vi "keithley-2450_sweep.vi"(4 "Timeout (ms)":i32=10000000, 5 "Scan direction":u16(ring) items=["Ascending", "Descending"], 6 "Number of Points":u32=5, 7 "End voltage (V)":dbl=2.0, 8 "Start voltage (V)":dbl=1.0, 9 "VISA resource name out 2":refnum<visa-resource-name>) -> (0 "Measurement Complete":bool, 2 "Data Array":dbl[][](array[numeric]), 3 "VISA resource name out":refnum<visa-resource-name>)   [LabVIEW 2016]
doc: "Configures a sweep and takes voltage and current readings at each point."
uses:
  <instrlib>/Keithley 2450/Keithley 2450.lvlib
panel:
  in  "Source Mode  (0: Voltage)":u16(ring) items=["Voltage", "Current"]
  # "(c) 2006 National Instruments.  ALL RIGHTS RESERVED."
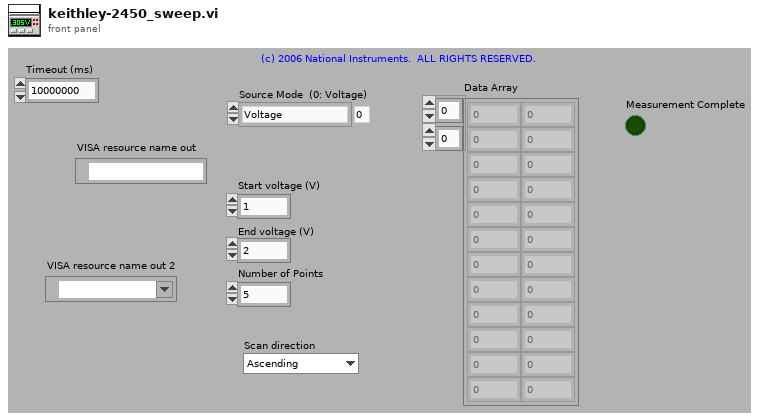
[diagram p1: front panel]
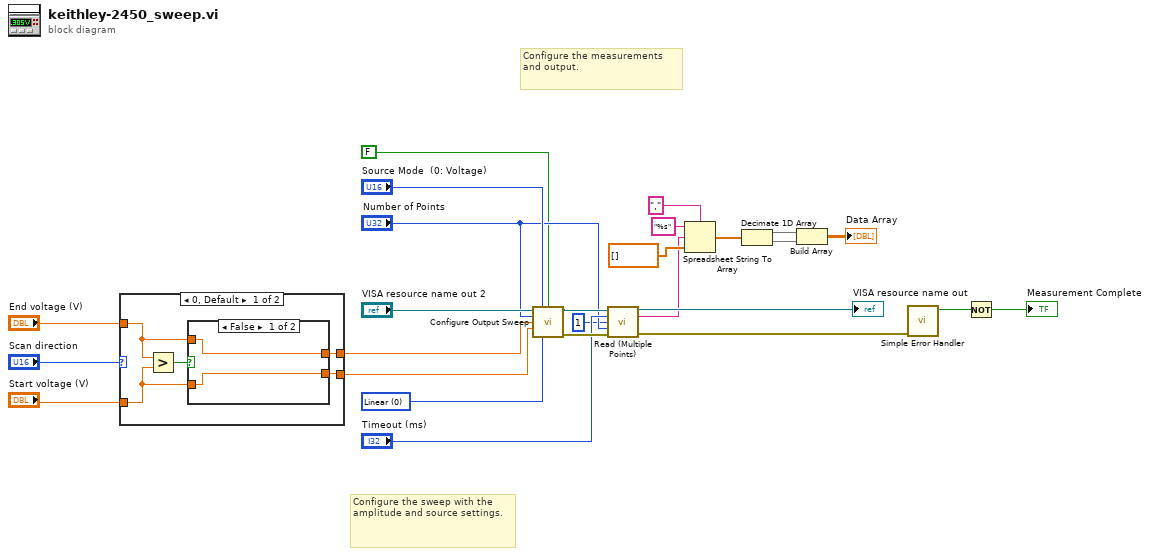
[diagram p0: block diagram]
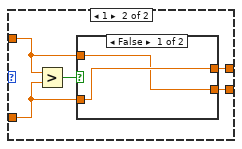
[diagram p3: hidden frame]
diagram:
  w17 = u16 0 items=["Linear", "Logarithmic"] ("Sweep Spacing  (0: Linear)")
  # "Configure the sweep with the amplitude and source settings."
  # "Configure the measurements and output."
  n1 = case shown="0, Default" "Scan direction" {
    tunnel: "End voltage (V)" -> [w28 w36]
    tunnel: "Start voltage (V)" -> [w30 w38]
    tunnel: [w29 w37] -> w2
    tunnel: [w27 w39] -> w1
    frame 0, Default {
      n2 = Greater?(x=w28, y=w30) -> (0:w31:bool)
      n3 = case shown="False" w31 {
        tunnel: [w32 w35] -> w29
        tunnel: w30 -> [w33 w35]
        tunnel: w28 -> [w32 w34]
        tunnel: [w33 w34] -> w27
        frame False {
        }
        frame True {
        }
      }
    }
    frame 1 {
      n4 = Greater?(x=w36, y=w38) -> (0:w40:bool)
      n5 = case shown="False" w40 {
        tunnel: [w41 w44] -> w39
        tunnel: w38 -> [w42 w44]
        tunnel: [w42 w43] -> w37
        tunnel: w36 -> [w41 w43]
        frame False {
        }
        frame True {
        }
      }
    }
  }
  n6 = call <instrlib>:"Configure Output Sweep.vi"("VISA resource name"="VISA resource name out 2", "Source Mode  (0: Voltage)"="Source Mode  (0: Voltage)", "Dual Sweep (F:Disable)"=FALSE, "Number of Points (5)"="Number of Points", "Start Amplitude (1)"=w2, "Stop Amplitude (2)"=w1, "Sweep Spacing  (0: Linear)"=w17) -> ("VISA resource name out"=w20:refnum<visa-resource-name>, "error out"=w19:errorcluster)  [unwired: 7 in]
  n7 = call <instrlib>:"Read (Multiple Points).vi"("VISA resource name"=w20, "Timeout (10000 ms)"="Timeout (ms)", "Start Index (1)"=u32 1, "End Index (1)"="Number of Points", "error in (no error)"=w19) -> ("VISA resource name out"=→"VISA resource name out":refnum<visa-resource-name>, "Data out"=w8:string, "error out"=w25:errorcluster)  [unwired: 8 in]
  n8 = Spreadsheet String To Array(delimiter (Tab)=",", format string="%s", spreadsheet string=w8, array type (2D Dbl)=dbl[] []) -> (array=w13:dbl[])
  n9 = Decimate 1D Array(w13) -> (w12:dbl[], w11:dbl[])
  n10 = Build Array(w12, w11) -> (→"Data Array":dbl[][])
  n11 = call <vilib>:"Simple Error Handler.vi"("error in (no error)"=w25) -> ("error?"=w23:bool)  [unwired: 4 in, 4 out]
  n12 = Not(x=w23) -> (.not. x?=→"Measurement Complete":bool)
